vi "4) Request Reply.vi"() -> ()   [LabVIEW 2020, in "VectoScratch.lvlib"]
uses:
  VectoScratch.lvlib
  Vecto/proto/TcpClientHello/Data.ctl
  RequestReply Message Handler/RequestReply Message Handler.lvclass
  C:/dev/lv20CE/relink/lv-vecto/Vecto/TCPMessageHandler/TCPMessageHandler.lvclass
  19c59f3d-4438-4bbc-9f5b-90826cadd21a.vi
  f43fa4b8-9013-4cdb-9f53-d6588b84612f.vi
  Vecto/TCPMessaging/TCPMessaging.lvclass
  Vecto/proto/TcpClientHello/TcpClientHello.lvlib
  Vecto/SequenceCountService/SequenceCountService.lvclass
  Vecto/TCPMessageService/TCPMessageAPI.lvclass
  proto/messages/RequestTwoDouble/RequestTwoDouble.lvlib
  proto/messages/ReplyOneDouble/ReplyOneDouble.lvlib
panel:
  out "Response":dbl
  in  "B":dbl=6.0
  in  "A":dbl=7.0
  out "Server Error":errorcluster
  out "Client Error":errorcluster
  # "Set A & B and then run the VI to perform multiplication via Request / Reply. The server sends the operands to the client and awaits the response."
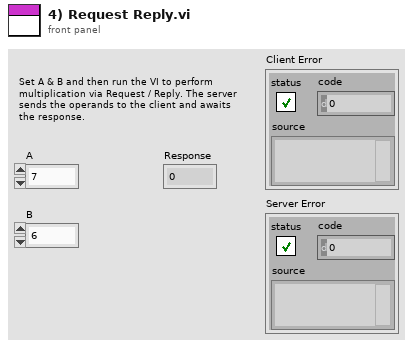
[diagram p1: front panel]
types:
  T1 = typedef "TcpClientHello.lvlib/Data.ctl" = cluster{"node_id":u32, "system":string, "cluster":string, "node_name":string, "app_version":string, "config_version":string}
  T2 = typedef "TcpPayload.lvlib/Data.ctl" = cluster{"target_node":u32, "source_id":u32, "sequence":u32, "timestamp":u64, "type":string, "task_id":string, "payload":u8[]}
  T3 = typedef "ReplyOneDouble.lvlib/Data.ctl" = cluster{"response":dbl}
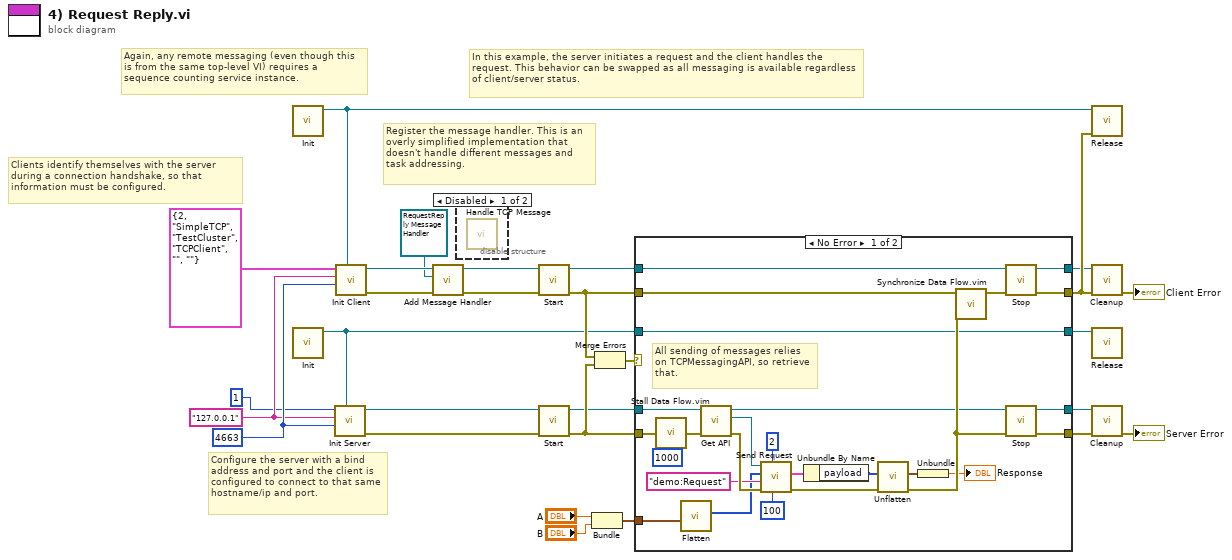
[diagram p0: block diagram]
diagram:
  w27 = u16 4663 ("Bind Port")
  w26 = "127.0.0.1" ("Bind Address")
  # "Register the message handler. This is an overly simplified implementation that doesn't handle different messages and task addressing."
  # "Clients identify themselves with the server during a connection handshake, so that information must be configured."
  # "Configure the server with a bind address and port and the client is configured to connect to that same hostname/ip and port."
  # "In this example, the server initiates a request and the client handles the request. This behavior can be swapped as all messaging is available regardless of client/server status."
  # "Again, any remote messaging (even though this is from the same top-level VI) requires a sequence counting service instance."
  n1 = call "Init.vi"() -> ("SequenceCountService out"=w11:refnum<class "SequenceCountService.lvclass">)  [unwired: 10 in, 1 out]
  n2 = call "Init.vi"() -> ("SequenceCountService out"=w2:refnum<class "SequenceCountService.lvclass">)  [unwired: 10 in, 1 out]
  n3 = call "Init Server.vi"("SequenceCountService"=w2, "Bind Port"=w27, "Bind Address"=w26, "Node ID"=u32 1) -> ("error out"=w3:errorcluster, "TCPMessaging out"=w4:refnum<class "TCPMessaging.lvclass">)  [unwired: 6 in]
  n4 = call "Init Client.vi"("SequenceCountService"=w11, "Remote Port"=w27, "Remote Address"=w26, "Client Info"=T1 {"node_id"=2, "system"="SimpleTCP", "cluster"="TestCluster", "node_name"="TCPClient", "app_version"="", "config_version"=""}) -> ("error out"=w9:errorcluster, "TCPMessaging out"=w10:refnum<class "TCPMessaging.lvclass">)  [unwired: 6 in]
  n5 = call "Add Message Handler.vi"("error in (no error)"=w9, "TCPMessageHandler"=refnum<class "RequestReply Message Handler.lvclass"> refnum ("VectoScratch.lvlib:RequestReply Message Handler.lvclass"), "TCPMessaging in"=w10) -> ("error out"=w23:errorcluster, "TCPMessaging out"=w24:refnum<class "TCPMessaging.lvclass">)  [unwired: 7 in]
  n6 = disable-structure shown="Disabled" {
    frame Disabled {
      n7 = call-dynamic "Handle TCP Message.vi"() -> ()  [unwired: 10 in, 2 out]
    }
    frame Enabled {
    }
  }
  n8 = call "Start.vi"("error in (no error)"=w23, "TCPMessaging in"=w24) -> ("error out"=w21:errorcluster, "TCPMessaging out"=w18:refnum<class "TCPMessaging.lvclass">)  [unwired: 8 in]
  n9 = call "Start.vi"("error in (no error)"=w3, "TCPMessaging in"=w4) -> ("error out"=w20:errorcluster, "TCPMessaging out"=w19:refnum<class "TCPMessaging.lvclass">)  [unwired: 8 in]
  n10 = Bundle("A"="A", "B"="B") -> (w5:cluster{"A":dbl, "B":dbl})  [unwired: 1 in]
  n11 = Merge Errors(w21, w20) -> (w22:errorcluster)
  n12 = case shown="No Error" w22 {
    tunnel: w21 -> [w44 w59]
    tunnel: w20 -> [w51 w58]
    tunnel: w19 -> [w52 w57]
    tunnel: w18 -> [w47 w56]
    tunnel: [w38 w59] -> w28
    tunnel: [w39 w58] -> w15
    tunnel: [w48 w57] -> w16
    tunnel: [w49 w56] -> w17
    tunnel: w5 -> [w34 _]
    tunnel: w2 -> [w35 w55]
    tunnel: [w35 w55] -> w1
    frame No Error {
      # "All sending of messages relies on TCPMessagingAPI, so retrieve that."
      n13 = call "Stall Data Flow.vim"("value in"=w51, "milliseconds to wait"=u32 1000) -> ("value out"=w41:errorcluster)  [unwired: 1 out]
      n14 = call "Flatten.vi"("Data"=w34) -> ("Buffer"=w33:u8[])  [unwired: 9 in, 1 out]
      n15 = call "Get API.vi"("error in (no error)"=w41, "TCPMessaging in"=w52) -> ("error out"=w53:errorcluster, "TCP Messaging API"=w46:refnum<class "TCPMessageAPI.lvclass">, "TCPMessaging out"=w50:refnum<class "TCPMessaging.lvclass">)  [unwired: 7 in]
      n16 = call "Send Request.vi"("Timeout mS (5000)"=100, "Target Node"=u32 2, "error in (no error)"=w53, "Type"="demo:Request", "Payload"=w33, "TCPMessageAPI in"=w46) -> ("error out"=w32:errorcluster, "Reply"=w42:T2)  [unwired: 3 in, 1 out]
      n17 = Unbundle By Name(w42) -> ("payload"=w31:u8[])
      n18 = call "Unflatten.vi"("error in"=w32, "Buffer"=w31) -> ("error out"=w54:errorcluster, "Data"=w30:T3)  [unwired: 8 in]
      n19 = Unbundle(w30) -> ("response"=→"Response":dbl)
      n20 = call "Synchronize Data Flow.vim"("input 4"=w54, "input 1"=w44) -> ("output 1"=w43:errorcluster)  [unwired: 2 in, 3 out]
      n21 = call "Stop.vi"("error in (no error)"=w43, "TCPMessaging in"=w47) -> ("error out"=w38:errorcluster, "TCPMessaging out"=w49:refnum<class "TCPMessaging.lvclass">)  [unwired: 8 in]
      n22 = call "Stop.vi"("error in (no error)"=w54, "TCPMessaging in"=w50) -> ("error out"=w39:errorcluster, "TCPMessaging out"=w48:refnum<class "TCPMessaging.lvclass">)  [unwired: 8 in]
    }
    frame Error {
    }
  }
  n23 = call "Release.vi"("error in (no error)"=w28, "SequenceCountService in"=w11) -> ()  [unwired: 9 in, 1 out]
  n24 = call "Cleanup.vi"("error in (no error)"=w28, "TCPMessaging in"=w17) -> ("error out"=→"Client Error":errorcluster)  [unwired: 9 in]
  n25 = call "Release.vi"("SequenceCountService in"=w1) -> ()  [unwired: 10 in, 1 out]
  n26 = call "Cleanup.vi"("error in (no error)"=w15, "TCPMessaging in"=w16) -> ("error out"=→"Server Error":errorcluster)  [unwired: 9 in]
